vi "Save TS Results.vi"(8 "error in":errorcluster, 11 "Test Stand in":refnum<class "Heat Flow Test Stand.lvclass">) -> (0 "error out":errorcluster, 3 "Test Stand out":refnum<class "Heat Flow Test Stand.lvclass">)   [LabVIEW 2019, in "Test Stands.lvlib" / "Heat Flow Test Stand.lvclass"]
uses:
  Heat Flow Test Stand.lvclass
  C:/Users/wg/Documents/LV_Projects/test-stand/App/Generic Test Stand/Generic Test Stand.lvclass
  Results/Results Method.ctl
  Generic Test Stand/Generic Test Stand.lvclass/Generic Test Stand.ctl
  DAC/DAC.lvclass
  Results/Results.lvlib
  Generic Test Stand/Generic Test Stand.lvclass
  Results/Heat Flow Results/Heat Flow Results.lvclass
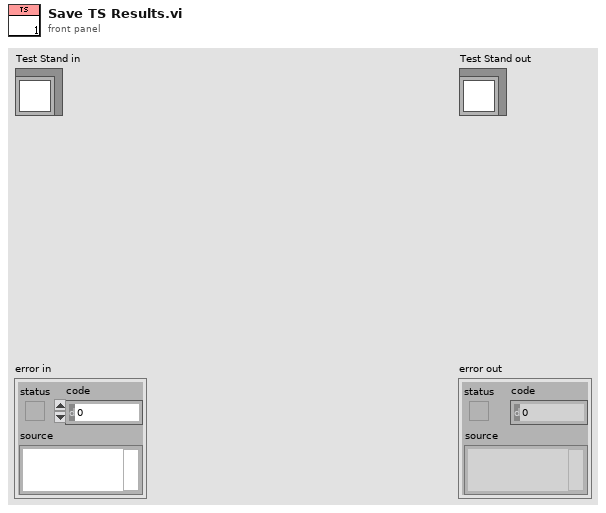
[diagram p1: front panel]
types:
  T1 = typedef "Results.lvlib/Results Method.ctl" = enum16{"Get", "Set"}
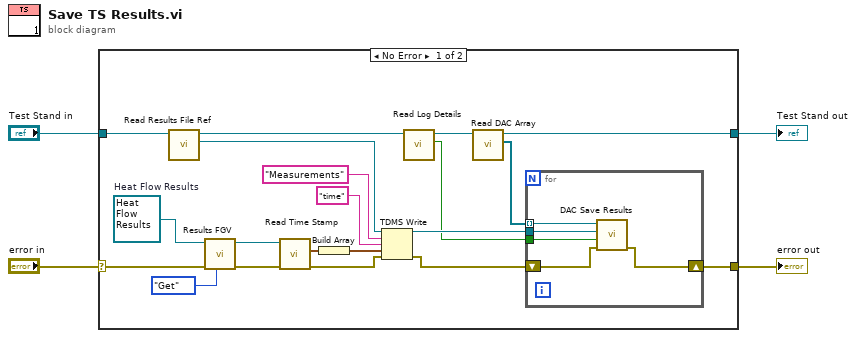
[diagram p0: block diagram]
diagram:
  n1 = case shown="No Error" "error in" {
    selector: "error in" -> [w16 w31]
    tunnel: "Test Stand in" -> [w23 w30]
    tunnel: [w12 w30] -> w2
    tunnel: [w9 w31] -> w1
    frame No Error {
      w5 = refnum<class "Heat Flow Results.lvclass"> refnum  # Heat Flow Results
      n2 = call "Read Results File Ref.vi"("Generic Test Stand in"=w23) -> ("Results File Ref"=w21:refnum<k34>, "Generic Test Stand out"=w8:refnum<class "Heat Flow Test Stand.lvclass">)  [unwired: 8 in, 1 out]
      n3 = call-dynamic "Results FGV.vi"("Method"=Results_Method."Get", "error in"=w16, "Results in"=w5) -> ("error out"=w15:errorcluster, "Results out"=w22:refnum<class "Heat Flow Results.lvclass">)  [unwired: 7 in]
      n4 = call-dynamic "Read Time Stamp.vi"("error in (no error)"=w15, "Results in"=w22) -> ("error out"=w14:errorcluster, "Time Stamp"=w20:timestamp)  [unwired: 7 in, 1 out]
      n5 = Build Array(w20) -> (w19:timestamp[])
      n6 = TDMS Write(0:w21, 5:"Measurements" ("group name in (Untitled)"), 7:"time" ("group name in (Untitled)"), 9:w19, 11:w14) -> (4:w13:refnum<k34>, 15:w10:errorcluster)  [unwired: 1 in, 2 out]
      n7 = call "Read Log Details.vi"("Generic Test Stand in"=w8) -> ("Log Details"=w6:bool, "Generic Test Stand out"=w7:refnum<class "Heat Flow Test Stand.lvclass">)  [unwired: 8 in, 1 out]
      n8 = call "Read DAC Array.vi"("Generic Test Stand in"=w7) -> ("DAC Array"=w11:refnum<class "DAC.lvclass">[], "Generic Test Stand out"=w12:refnum<class "Heat Flow Test Stand.lvclass">)  [unwired: 8 in, 1 out]
      n9 = for {
        tunnel: w11 -> [w29] mode=indexing
        shift-right: [w26] -> w9
        shift-left: w10 -> [w27]
        tunnel: w13 -> [w28]
        tunnel: w6 -> [w25]
        n10 = call-dynamic "DAC Save Results.vi"("error in"=w27, "Log Details?"=w25, "tdms file"=w28, "DAC in"=w29) -> ("error out"=w26:errorcluster)  [unwired: 7 in]
      }
    }
    frame Error {
    }
  }
  "error out" <- w1
  "Test Stand out" <- w2
